vi "ex5-5.vi"() -> ()   [LabVIEW 2014]
uses:
  <vilib>/NXT/Dual Mode Library/Motors/MotorOn.vi
  <vilib>/NXT/Dual Mode Library/Waits/Wait_Rotation.vi
  <vilib>/NXT/Dual Mode Library/Motors/MotorCoast.vi
  <vilib>/express/express arith-compare/Formula/XNode/ExpressFormulaBlockNode.xnode
panel:
  in  "行進距離(cm)":dbl
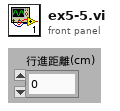
[diagram p1: front panel]
types:
  T1 = typedef "LVHSConnector.ctl" = refnum<class "BrickReference.lvclass">
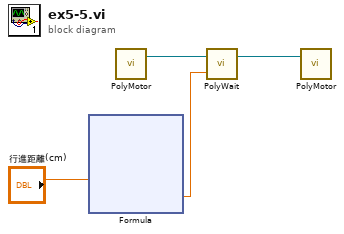
[diagram p0: block diagram]
diagram:
  n1 = xnode "Formula"("X1"="行進距離(cm)") -> ("Result"=w3:dbl)  [unwired: 1 in, 1 out]
  n2 = call-poly <vilib>:"PolyMotor.vi"() -> ("NXT/EV3"=w1:T1)  [unwired: 4 in]
  n3 = call-poly <vilib>:"PolyWait.vi"("Position Change (180)"=w3, "NXT/EV3"=w1) -> ("NXT/EV3"=w2:T1)  [unwired: 2 in]
  n4 = call-poly <vilib>:"PolyMotor.vi"("NXT/EV3"=w2) -> ()  [unwired: 3 in, 1 out]
